vi "PH_BeamlineController.get Source Attributes.vi"(0 "VI in":refnum<vi>, 2 "Source":T1, 5 "error in (no error)":errorcluster) -> (14 "VI out":refnum<vi>, 17 "Source Index":i32, 18 "Source Attributes":T2, 19 "error out":errorcluster)   [LabVIEW 2014, in "PH_BeamlineController.lvlib"]
uses:
  PH_BeamlineController.lvlib
  PH_BeamlineController.Source Attributes.ctl
  PH_BeamlineController.Sources.ctl
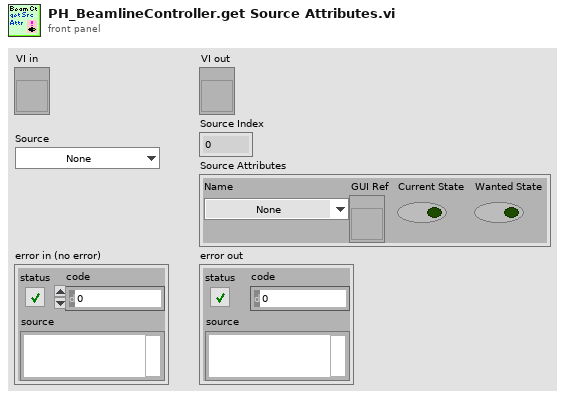
[diagram p1: front panel]
types:
  T1 = typedef "PH_BeamlineController.lvlib/PH_BeamlineController.Sources.ctl" = enum16{"None", "YLF", "fs-Frontend", "ns-Frontend", "YLF and ns-Frontend", "fs- and ns-Frontend"}
  T2 = typedef "PH_BeamlineController.lvlib/PH_BeamlineController.Source Attributes.ctl" = cluster{"Name":T1, "GUI Ref":refnum<vi>, "Current State":bool, "Wanted State":bool}
  T3 = typedef "PH_BeamlineController.lvlib/PH_BeamlineController.i attribute.ctl" = cluster{"Vacuum Exp LB":cluster{"Channel":string, "Limit [mbar]":dbl, "Pressure [mbar]":dbl, "GUI Ref":refnum<vi>}, "Sources":T2[], "PA DP Targets":T4[], "Path":cluster{"Source":T1, "PA DP Target":T5, "Target":T6}, "Targets":cluster{"Name":T6, "GUI Ref":refnum<vi>, "Current State":bool, "Wanted State":bool, "Enabled":bool}[], "Status Tags":cluster{"Name":string, "Status":T7}[], "special GUI Refs":T8}
  T4 = typedef "PH_BeamlineController.lvlib/PH_BeamlineController.PA DP Target Attributes.ctl" = cluster{"Name":T5, "GUI Ref":refnum<vi>, "Current State":bool, "Wanted State":bool, "Enabled":bool}
  T5 = typedef "PH_BeamlineController.lvlib/PH_BeamlineController.PA DP Targets.ctl" = enum16{"None", "Dump PA Delayed Beam", "Dump PA Undelayed Beam", "Dumps PA Delayed and Undelayed Beam"}
  T6 = typedef "PH_BeamlineController.lvlib/PH_BeamlineController.Targets.ctl" = enum16{"None", "PreAmp", "Dump Exp Laserlab", "Exp Laserlab", "Calorimeter", "Dump Exp Laserbay", "Exp Laserbay", "Dump Exp Z6", "Exp Z6"}
  T7 = typedef "PH_StatusHandler.lvlib/PH_StatusHandler.Status.ctl" = i16
  T8 = typedef "PH_BeamlineController.lvlib/PH_BeamlineController.special GUI Refs.ctl" = cluster{"PA-Backreflection-Meas":refnum<vi>, "fs_Synchrolock_Watch":refnum<vi>}
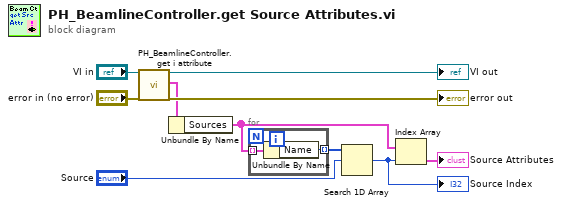
[diagram p0: block diagram]
diagram:
  n1 = call "PH_BeamlineController.get i attribute.vi"("i ref in"="VI in", "error in (no error)"="error in (no error)") -> ("i ref out"=→"VI out":refnum<vi>, "i attribute"=w4:T3, "error out"=→"error out":errorcluster)  [unwired: 15 in]
  n2 = Unbundle By Name(w4) -> ("Sources"=w2:T2[])
  n3 = for {
    tunnel: w2 -> [w12] mode=indexing
    tunnel: [w11] -> w1 mode=indexing
    n4 = Unbundle By Name(w12) -> ("Name"=w11:T1)
  }
  n5 = Search 1D Array(1D array=w1, element="Source") -> (index of element=w3:i32)  [unwired: 1 in]
  "Source Index" <- w3
  n6 = Index Array(array=w2, index=w3) -> (element=→"Source Attributes":T2)
